vi "PSTR-Repair Data File.vi"(0 "Data in":T11, 5 "path":path, 7 "PSTR Params":T2={"Stimulus"={"Ear"=enum."Right", "BW (oct)"=0.25, "Seed"=37, "Ramp (ms)"=5.0, "On time (ms)"=300.0, "Off time (ms)"=300.0, "Delay (ms)"=10000.0}, "FreqSeq"={"Min (kHz)"=4.0, "Max (kHz)"=64.0, "Step (oct)"=0.5}, "LevelSeq"={"Min (dB)"=0.0, "Max (dB)"=80.0, "Step (dB)"=20.0}, "Seq"={"Order"=enum."Sequential", "Averages"=20}, "Response"={"Grass gain"=10000.0, "Window (ms)"=0.0}, "Hidden"={"Sample rate (Hz)"=200000.0, "Nfft"=0, "save raw"=FALSE, "sep"=0.0, "Window"=enum."NONE"}, "RejThr"=0.0}, 9 "CFTS-PSTR":T1, 11 "error in (no error)":errorcluster) -> (4 "Data out":T11, 15 "error out":errorcluster)   [LabVIEW 2020]
uses:
  Typedefs/PSTR-Data.ctl
  Typedefs/PSTR-Model Fit.ctl
  Typedefs/PSTR-Fit Parameters.ctl
  Typedefs/PSTR-Parameters.ctl
  Typedefs/PSTR-Stimulus Params.ctl
  Utility VIs/Type Defs/Left-Right ring.ctl
  Typedefs/PSTR-FreqSeq Params.ctl
  Typedefs/PSTR-LevelSeq Params.ctl
  Typedefs/PSTR-SeqParams.ctl
  Typedefs/PSTR-Response Params.ctl
  Typedefs/PSTR-Hidden Params.ctl
  Typedefs/PSTR-Window Shape.ctl
  Typedefs/PSTR-File Info.ctl
panel:
  # "Fixing PSTRs and recomputing double-exponential fits..."
  # "NF x NL x 2 x Npts"
  # "NF x NL x Npts"
  # "NF x NL"
  # "NF x NL x 2 x Npts"
  # "NF x NL x Npts"
  # "NF x NL"
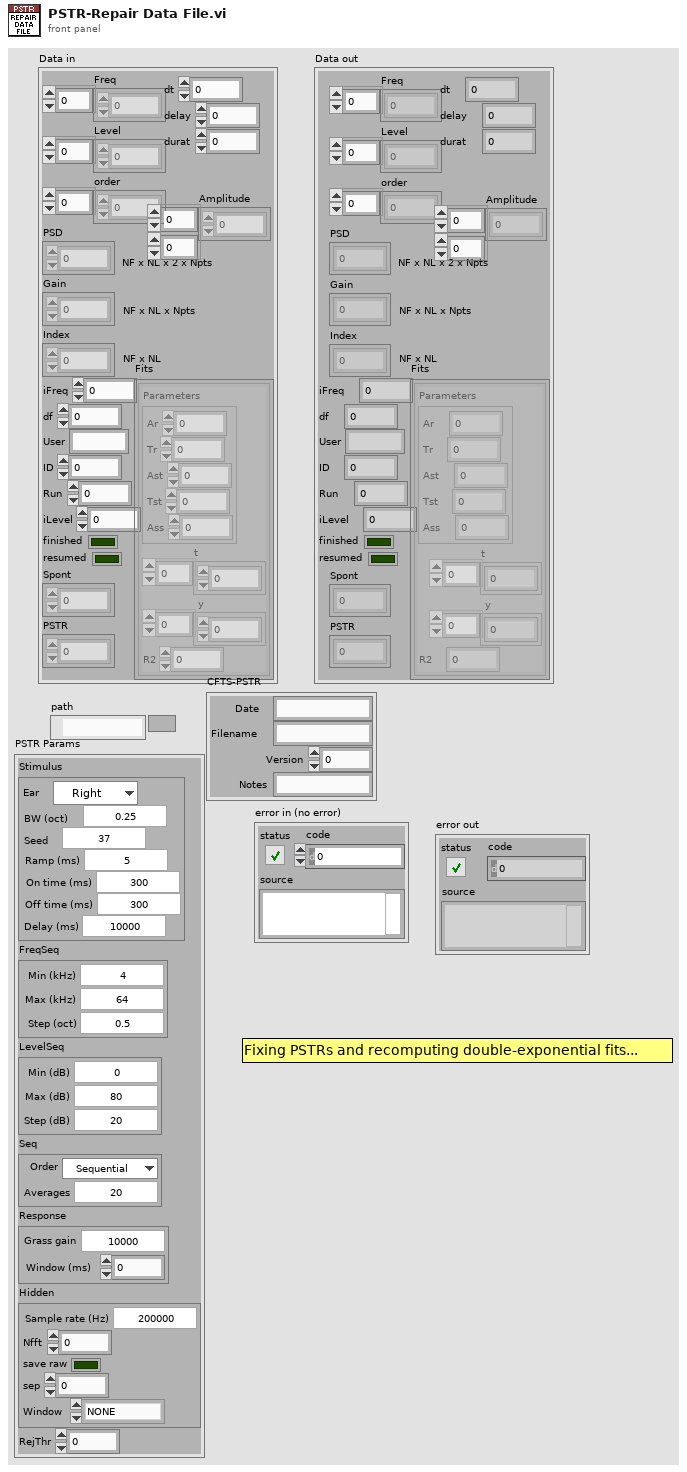
[diagram p1: front panel]
types:
  T1 = typedef "PSTR-File Info.ctl" = cluster{"Date":string, "Filename":string, "Version":i32, "Notes":string}
  T2 = typedef "PSTR-Parameters.ctl" = cluster{"Stimulus":T3, "FreqSeq":T5, "LevelSeq":T6, "Seq":T7, "Response":T8, "Hidden":T9, "RejThr":dbl}
  T3 = typedef "PSTR-Stimulus Params.ctl" = cluster{"Ear":T4, "BW (oct)":dbl, "Seed":i32, "Ramp (ms)":dbl, "On time (ms)":dbl, "Off time (ms)":dbl, "Delay (ms)":dbl}
  T4 = typedef "Left-Right ring.ctl" = enum16{"Right", "Left"}
  T5 = typedef "PSTR-FreqSeq Params.ctl" = cluster{"Min (kHz)":dbl, "Max (kHz)":dbl, "Step (oct)":dbl}
  T6 = typedef "PSTR-LevelSeq Params.ctl" = cluster{"Min (dB)":dbl, "Max (dB)":dbl, "Step (dB)":dbl}
  T7 = typedef "PSTR-SeqParams.ctl" = cluster{"Order":enum16{"Sequential", "Random"}, "Averages":i32}
  T8 = typedef "PSTR-Response Params.ctl" = cluster{"Grass gain":dbl, "Window (ms)":dbl}
  T9 = typedef "PSTR-Hidden Params.ctl" = cluster{"Sample rate (Hz)":dbl, "Nfft":i32, "save raw":bool, "sep":dbl, "Window":T10}
  T10 = typedef "PSTR-Window Shape.ctl" = enum16{"NONE", "Hamming"}
  T11 = typedef "PSTR-Data.ctl" = cluster{"Freq":dbl[], "Level":dbl[], "order":i32[], "PSD":dbl[][][][], "Gain":dbl[][][], "Index":dbl[][], "iFreq":i32, "df":dbl, "User":string, "ID":i32, "Run":i32, "iLevel":i32, "finished":bool, "resumed":bool, "Spont":dbl[][], "PSTR":dbl[][][], "dt":dbl, "delay":dbl, "durat":dbl, "Fits":T12[][], "Amplitude":dbl[][]}
  T12 = typedef "PSTR-Model Fit.ctl" = cluster{"Parameters":T13, "t":dbl[], "y":dbl[], "R2":dbl}
  T13 = typedef "PSTR-Fit Parameters.ctl" = cluster{"Ar":dbl, "Tr":dbl, "Ast":dbl, "Tst":dbl, "Ass":dbl}
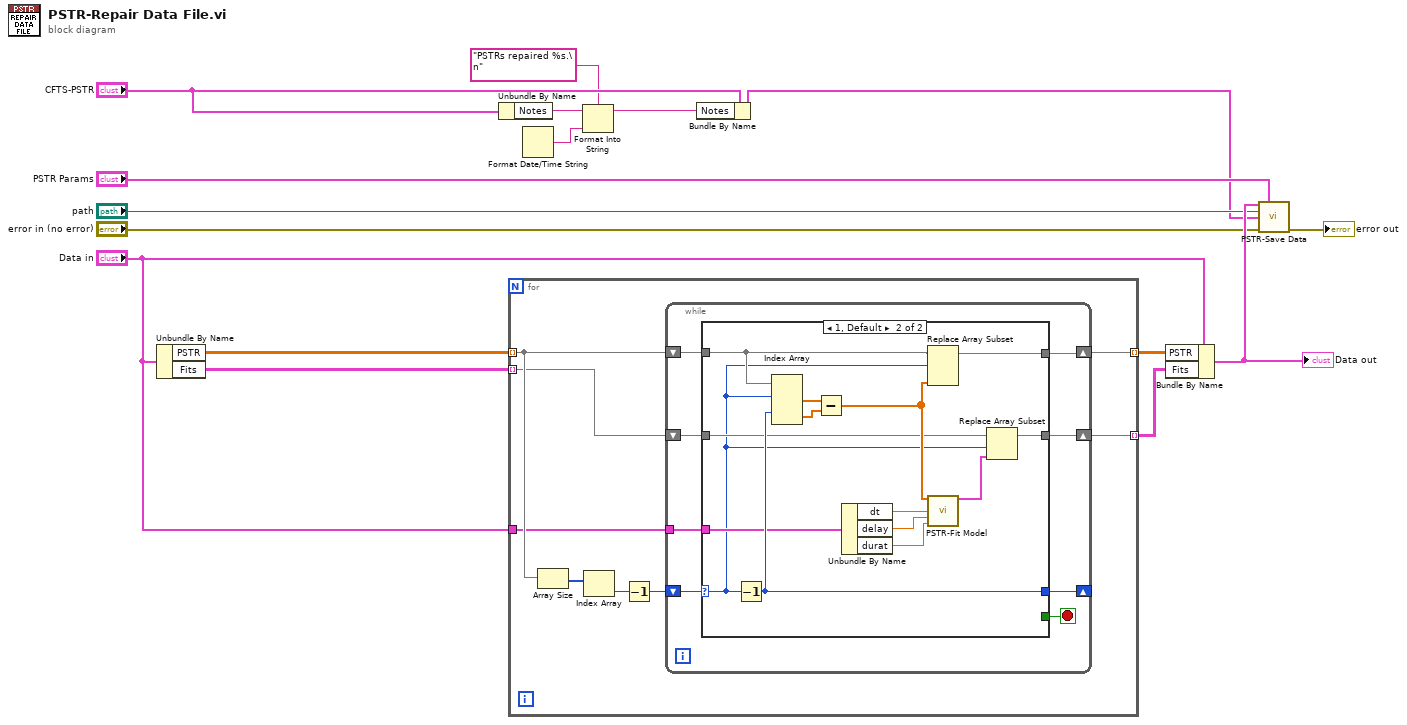
[diagram p0: block diagram]
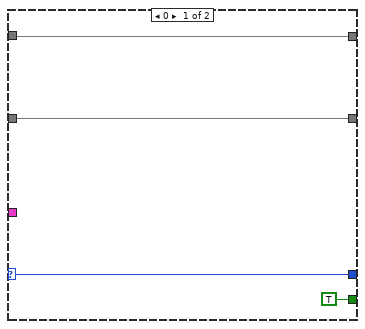
[diagram p2: hidden frame]
diagram:
  n1 = Unbundle By Name("Data in") -> ("PSTR"=w16:dbl[][][], "Fits"=w15:T12[][])
  n2 = Unbundle By Name("CFTS-PSTR") -> ("Notes"=w4:string)
  n3 = for {
    tunnel: w16 -> [w24] mode=indexing
    tunnel: w15 -> [w20] mode=indexing
    tunnel: "Data in" -> [w19]
    tunnel: [w18] -> w6 mode=indexing
    tunnel: [w17] -> w5 mode=indexing
    n4 = Array Size(array=w24) -> (size(s)=w23:i32[])
    n5 = Index Array(array=w23) -> (element=w22:i32)  [unwired: 1 in]
    n6 = Decrement(x=w22) -> (x-1=w21:i32)
    n7 = while {
      shift-right: [w30] -> _
      shift-left: w21 -> [w31]
      tunnel: w19 -> [w27]
      shift-right: [w26] -> w18
      shift-left: w24 -> [w32]
      shift-right: [w25] -> w17
      shift-left: w20 -> [w28]
      stop <- w29 stop-if-true
      n8 = case shown="1, Default" w31 {
        selector: w31 -> [w36 w39]
        tunnel: w32 -> [w34 w43]
        tunnel: [w36 w50] -> w30
        tunnel: [TRUE _] -> w29
        tunnel: w28 -> [w33 w40]
        tunnel: w27 -> [_ w44]
        tunnel: [w34 w42] -> w26
        tunnel: [w33 w38] -> w25
        frame 0 {
        }
        frame 1, Default {
          n9 = Decrement(x=w39) -> (x-1=w50:i32)
          n10 = Index Array(array=w43, index (row) #1=w39, index (row) #2=w50) -> (element #1=w49:dbl[], element #2=w48:dbl[])  [unwired: 2 in]
          n11 = Subtract(x=w49, y=w48) -> (x-y=w41:dbl[])
          n12 = Unbundle By Name(w44) -> ("dt"=w47:dbl, "delay"=w45:dbl, "durat"=w46:dbl)
          n13 = Replace Array Subset(array=w43, new element=w41, index (row)=w39) -> (w42:dbl[][])  [unwired: 1 in]
          n14 = call "PSTR-Fit Model.vi"("PSTH"=w41, "dt (ms)"=w47, "delay (ms)"=w45, "durat (ms)"=w46) -> ("Fit"=w37:T12)  [unwired: 11 in]
          n15 = Replace Array Subset(array=w40, new element=w37, index=w39) -> (w38:T12[])
        }
      }
    }
  }
  n16 = Format Date/Time String() -> (date/time string=w1:string)  [unwired: 3 in]
  n17 = Format Into String(format string="PSTRs repaired %s.\n", initial string=w4, w1) -> (resulting string=w3:string)  [unwired: 1 in, 1 out]
  n18 = Bundle By Name(cluster="CFTS-PSTR", "Notes"=w3) -> (w10:T1)
  n19 = Bundle By Name(cluster="Data in", "PSTR"=w6, "Fits"=w5) -> (w13:T11)
  "Data out" <- w13
  n20 = call "PSTR-Save Data.vi"("Data in"=w13, "PSTR Params"="PSTR Params", "path"="path", "CFTS-PSTR"=w10, "error in"="error in (no error)") -> ("Error Out"=→"error out":errorcluster)  [unwired: 8 in, 2 out]
